vi "Entry.vi"(8 "error in (no error)":errorcluster, 11 "Start Delay in":refnum<class "Start Delay.lvclass">) -> (0 "error out":errorcluster, 3 "Start Delay out":refnum<class "Start Delay.lvclass">)   [LabVIEW 2024, in "Sample State Actor.lvlib" / "Start Delay.lvclass"]
uses:
  Start Delay.lvclass
  C:/Program Files (x86)/National Instruments/LabVIEW 2024/vi.lib/ActorFramework/Actor/Actor.lvclass
  State Actor Messages/Delay Complete Msg/Delay Complete Msg.lvclass
  C:/Program Files (x86)/National Instruments/LabVIEW 2024/vi.lib/ActorFramework/Message/Message.lvclass
  <vilib>/ActorFramework/Actor/Actor.lvclass/Actor.ctl
  <vilib>/ActorFramework/Message Enqueuer/Message Enqueuer.lvclass/Message Enqueuer.ctl
  <vilib>/ActorFramework/Message Enqueuer/Init from Existing Queue.vi
  <vilib>/ActorFramework/Message Enqueuer/Message Enqueuer.lvclass
  Start Delay.lvclass/Start Delay.ctl
  <vilib>/ActorFramework/Actor/Actor.lvclass
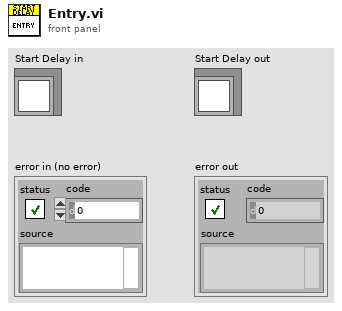
[diagram p1: front panel]
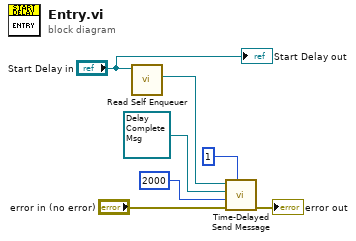
[diagram p0: block diagram]
diagram:
  n1 = call <vilib>:"Read Self Enqueuer.vi"("Actor"="Start Delay in") -> ("Self Enqueuer"=w7:refnum<class "Message Enqueuer.lvclass">)  [unwired: 10 in]
  n2 = call <vilib>:"Time-Delayed Send Message.vi"("# Copies (0 = infinite repeat)"=u32 1, "error in (no error)"="error in (no error)", "Milliseconds To Wait"=2000, "Message"=refnum<class "Delay Complete Msg.lvclass"> refnum ("State Actor.lvlib:Delay Complete Msg.lvclass"), "Message Enqueuer"=w7) -> ("error out"=→"error out":errorcluster)  [unwired: 5 in, 1 out]
  "Start Delay out" <- "Start Delay in"
